vi "SaveCalibrationFile(SubVI).vi"(3 "System ID":string(combo), 4 "V2":dbl, 5 "Ch1 Data":dbl[](array[numeric]), 6 "V1":dbl, 7 "appended path":path, 8 "error in (no error)":errorcluster, 9 "Ch3 Data":dbl[](array[numeric]), 10 "V3":dbl, 11 "Ch2 Data":dbl[](array[numeric])) -> (0 "error out":errorcluster)   [LabVIEW 2024]
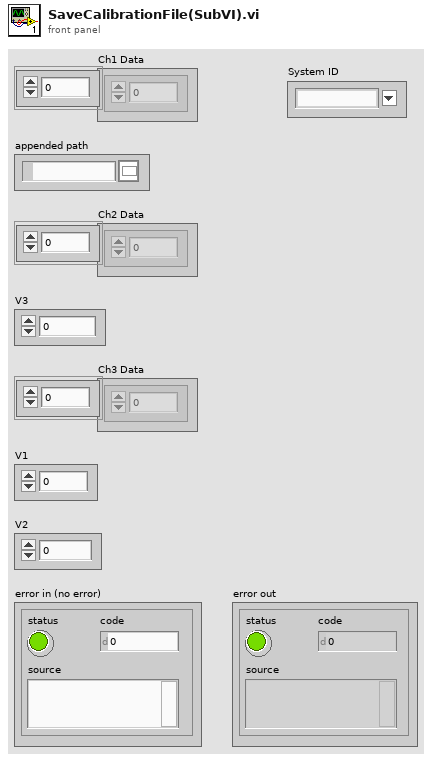
[diagram p1: front panel]
types:
  T1 = enum16{"open", "open or create", "create or replace", "create", "open (read-only)"}
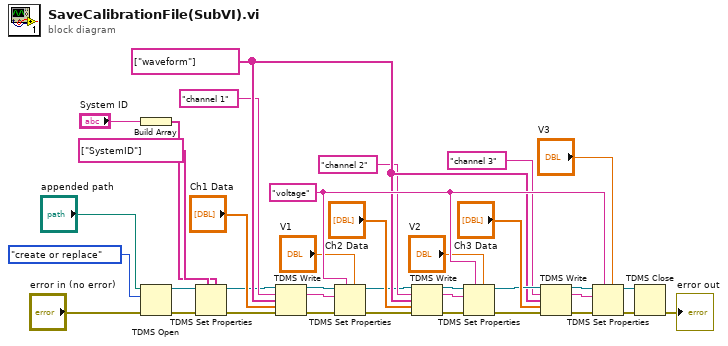
[diagram p0: block diagram]
diagram:
  w35 = "voltage" ("property names")
  w28 = string[] ["waveform"] ("channel name(s) in (Untitled)")
  n1 = Build Array("System ID") -> (w1:string[])
  n2 = TDMS Open(8:"error in (no error)", 10:T1."create or replace" ("operation (0:open)"), 11:"appended path") -> (0:w5:errorcluster, 3:w7:refnum<k34>)  [unwired: 4 in]
  n3 = TDMS Set Properties(5:w1, 7:string[] ["SystemID"] ("property names"), 8:w5, 11:w7) -> (0:w4:errorcluster, 3:w6:refnum<k34>)  [unwired: 2 in, 2 out]
  n4 = TDMS Write(0:w6, 5:"channel 1" ("group name in (Untitled)"), 7:w28, 9:"Ch1 Data", 11:w4) -> (4:w11:refnum<k34>, 6:w21:string, 15:w12:errorcluster)  [unwired: 1 in, 1 out]
  n5 = TDMS Set Properties(5:"V1", 7:w35, 8:w12, 10:w21, 11:w11) -> (0:w18:errorcluster, 3:w17:refnum<k34>)  [unwired: 1 in, 2 out]
  n6 = TDMS Write(0:w17, 5:"channel 2" ("group name in (Untitled)"), 7:w28, 9:"Ch2 Data", 11:w18) -> (4:w22:refnum<k34>, 6:w23:string, 15:w24:errorcluster)  [unwired: 1 in, 1 out]
  n7 = TDMS Set Properties(5:"V2", 7:w35, 8:w24, 10:w23, 11:w22) -> (0:w26:errorcluster, 3:w29:refnum<k34>)  [unwired: 1 in, 2 out]
  n8 = TDMS Write(0:w29, 5:"channel 3" ("group name in (Untitled)"), 7:w28, 9:"Ch3 Data", 11:w26) -> (4:w31:refnum<k34>, 6:w33:string, 15:w32:errorcluster)  [unwired: 1 in, 1 out]
  n9 = TDMS Set Properties(5:"V3", 7:w35, 8:w32, 10:w33, 11:w31) -> (0:w37:errorcluster, 3:w36:refnum<k34>)  [unwired: 1 in, 2 out]
  n10 = TDMS Close(8:w37, 11:w36) -> (0:→"error out":errorcluster)  [unwired: 1 out]
